vi "Destroy Message Queue.vi"(0 "message queue in":T3, 11 "error in":errorcluster) -> (4 "message queue name":string, 6 "remaining elements":T1[](array[typedef]), 15 "error out":errorcluster)   [LabVIEW 2012, in "Car Wash.lvlib" / "AMC.lvlib"]
doc: "Releases the reference to the message queue and returns any remaing messages."
uses:
  AMC.lvlib
  Message Queue.ctl
  Message.ctl
  Tools/Keyed Array/KeyedArray.ctl
  Queue Registry Method.ctl
  Tools/Keyed Array/Tools_KeyedArray.lvlib
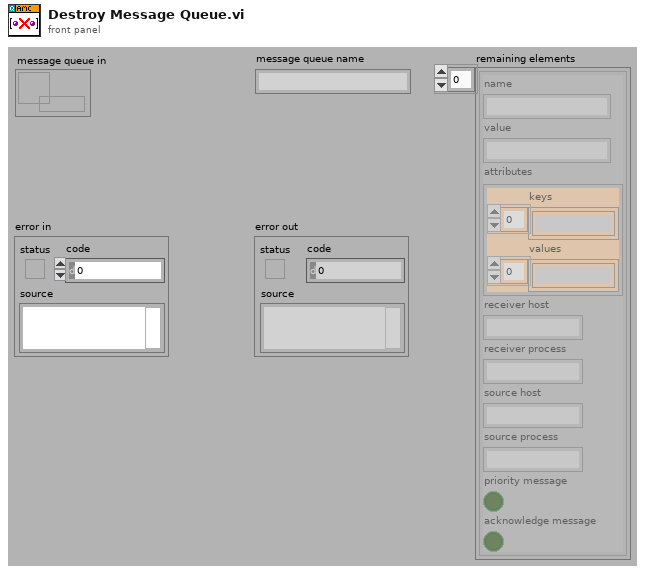
[diagram p1: front panel]
types:
  T1 = typedef "Car Wash.lvlib/AMC.lvlib/Message.ctl" = cluster{"name":string, "value":string, "attributes":T2, "receiver host":string, "receiver process":string, "source host":string, "source process":string, "priority message":bool, "acknowledge message":bool}
  T2 = typedef "Car Wash.lvlib/Tools_KeyedArray.lvlib/KeyedArray.ctl" = cluster{"keys":string[], "values":string[]}
  T3 = typedef "Car Wash.lvlib/AMC.lvlib/Message Queue.ctl" = refnum<queue>
  T4 = typedef "Car Wash.lvlib/AMC.lvlib/Queue Registry Method.ctl" = enum16{"Initialize", "Add Queue", "Set Properties", "Get Queue by Index", "Get Queue by Name", "Remove Queue", "Remove All Queues"}
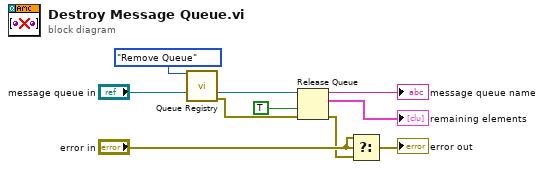
[diagram p0: block diagram]
diagram:
  n1 = call "Queue Registry.vi"("method"=Queue_Registry_Method."Remove Queue" ("Method"), "message queue in"="message queue in") -> ("message queue out"=w6:T3, "error out"=w5:errorcluster)  [unwired: 8 in, 4 out]
  n2 = Release Queue(queue=w6, force destroy? (F)=TRUE, error in (no error)=w5) -> (queue name=→"message queue name":string, remaining elements=→"remaining elements":T1[], error out=w2:errorcluster)
  n3 = Select(t="error in", s="error in", f=w2) -> (s? t:f=→"error out":errorcluster)
